vi "Target Angle (Set).vi"(6 "ISOBUS address":T4=-1 caption="ISOBUS address (-1)", 8 "error in":errorcluster, 9 "Unit":T2, 10 "Position":dbl, 11 "Mercury Reference In":T5) -> (0 "error out":errorcluster, 2 "Response":T1, 3 "Mercury Reference Out":T5, 4 "Valid?":T3)   [LabVIEW 2019, in "Mercury iXX.lvlib" / "Auxiliary.lvlib"]
doc: "Acquire the current position of the stepper motor."
uses:
  Auxiliary.lvlib
  Controls/Mercury Reference.ctl
  Controls/Comms Transport Layer.ctl
  Private/Controls/Query Dynamic Reference.ctl
  Controls/ISOBus Address.ctl
  Controls/Is Valid LED.ctl
  Controls/Unit String.ctl
  Controls/Response String.ctl
  Private/Controls/Command Verbs.ctl
  Mercury iXX.lvlib
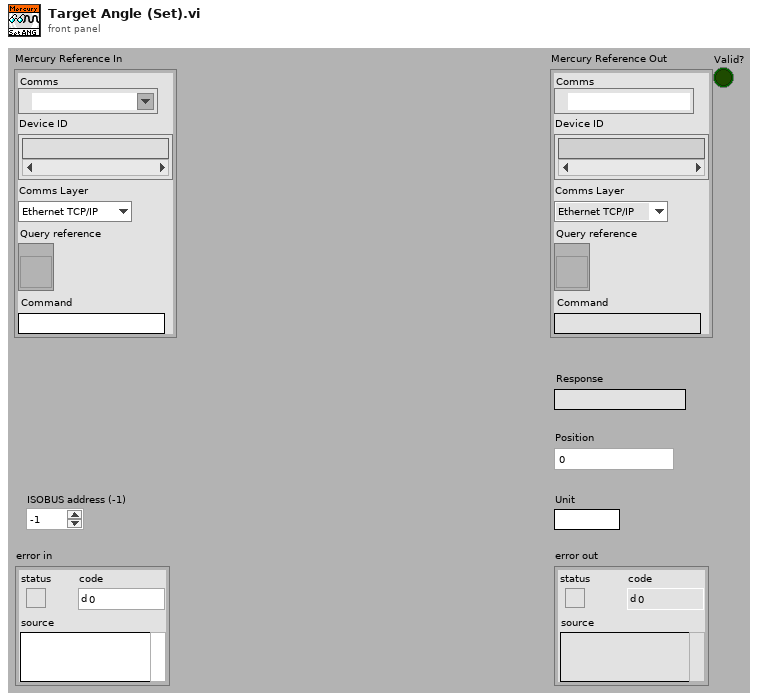
[diagram p1: front panel]
types:
  T1 = typedef "Mercury iXX.lvlib/Response String.ctl" = string
  T2 = typedef "Mercury iXX.lvlib/Unit String.ctl" = string
  T3 = typedef "Mercury iXX.lvlib/Is Valid LED.ctl" = bool
  T4 = typedef "Mercury iXX.lvlib/ISOBus Address.ctl" = i32
  T5 = typedef "Mercury iXX.lvlib/Mercury Reference.ctl" = cluster{"Comms":refnum<visa-resource-name>, "Device ID":string[], "Comms Layer":T6, "Command":string, "Query reference":T7}
  T6 = typedef "Mercury iXX.lvlib/Comms Transport Layer.ctl" = enum16{"Ethernet TCP/IP", "USB", "ISOBus - RS-232", "GPIB"}
  T7 = typedef "Mercury iXX.lvlib/Query Dynamic Reference.ctl" = refnum<vi>
  T8 = typedef "Mercury iXX.lvlib/Command Verbs.ctl" = string
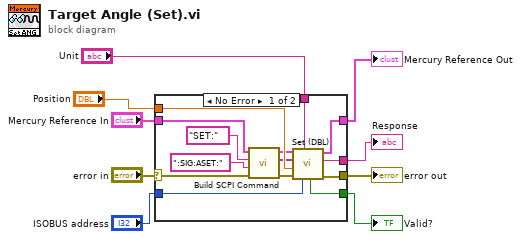
[diagram p0: block diagram]
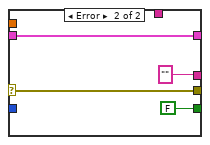
[diagram p2: hidden frame]
diagram:
  n1 = case shown="No Error" "error in" {
    selector: "error in" -> [w22 w26]
    tunnel: "Mercury Reference In" -> [w23 w27]
    tunnel: [w16 w26] -> w4
    tunnel: [w12 w27] -> w6
    tunnel: "ISOBUS address" -> [w18 _]
    tunnel: [w19 T3 FALSE ("Valid?")] -> w5
    tunnel: "Position" -> [w15 _]
    tunnel: "Unit" -> [w11 _]
    tunnel: [w10 T1 "" ("Response")] -> w1
    frame No Error {
      n2 = call "Build SCPI Command.vi"("error in"=w22, "Noun(s)"=":SIG:ASET:" ("Command"), "Verb"=T8 "SET:", "Mercury Reference In"=w23) -> ("error out"=w17:errorcluster, "SCPI Message(s)"=w14:string[], "Mercury Reference Out"=w13:T5)  [unwired: 5 out]
      n3 = call "Set (DBL).vi"("ISOBUS address"=w18, "Unit"=w11, "error in"=w17, "Command Value (Dbl)"=w15, "SCPI Message(s)"=w14, "Mercury Reference In"=w13) -> ("error out"=w16:errorcluster, "Response"=w10:T1, "Mercury Reference Out"=w12:T5, "Valid?"=w19:T3)  [unwired: 2 in]
    }
    frame Error {
    }
  }
  "Mercury Reference Out" <- w6
  "Valid?" <- w5
  "error out" <- w4
  "Response" <- w1
